vi "Generarea si afisarea grafica simultana a mai multor semnale.vi"() -> ()   [LabVIEW 2011]
uses:
  <vilib>/measure/NI_MABase.lvlib
panel:
  in  "Phase 2":dbl
  in  "Amplitude 2":dbl
  in  "Frequency 2":dbl
  in  "Sampling 2":cluster{"Fs":dbl, "#s":dbl}
  in  "Reset phase 2":bool
  in  "Reset phase":bool
  out "Waveform Graph":waveform(dbl)[](graph)
  out "error out":errorcluster
  in  "Sampling":cluster{"Fs":dbl, "#s":dbl}
  in  "Frequency":dbl
  in  "Amplitude":dbl
  in  "Phase":dbl
  in  "stop":bool
  out "error out 2":errorcluster
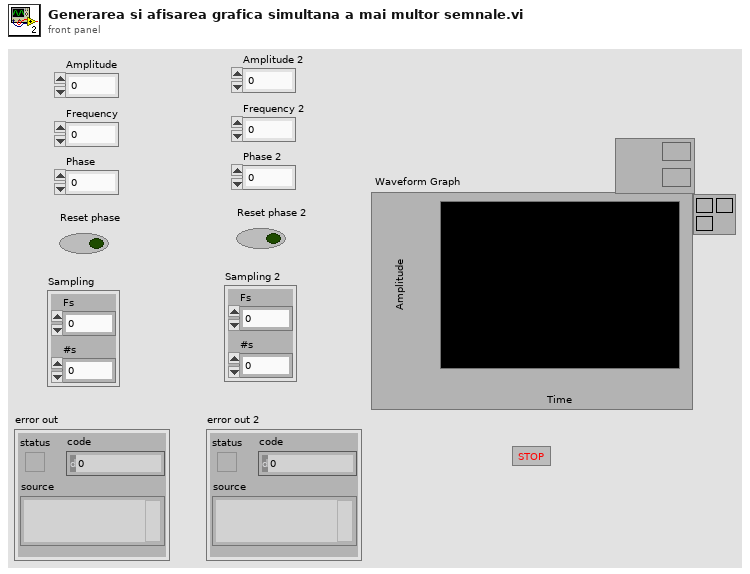
[diagram p1: front panel]
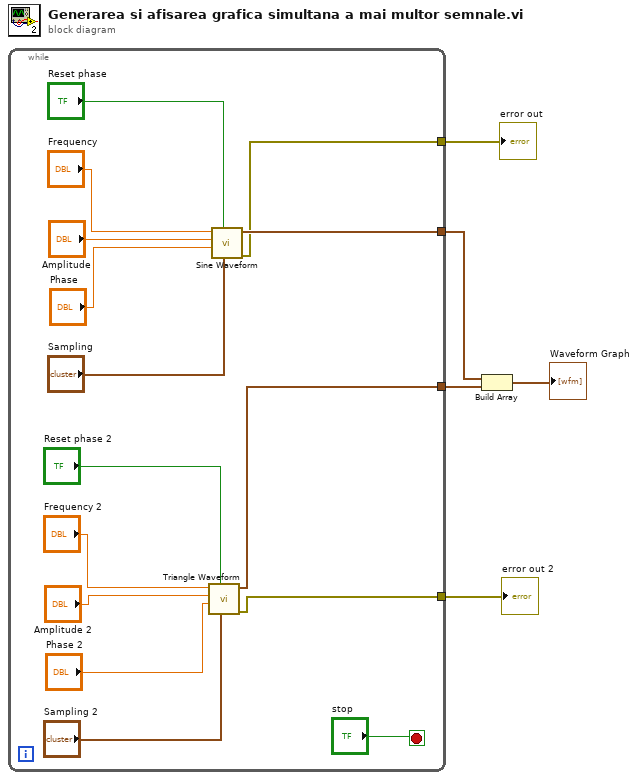
[diagram p0: block diagram]
diagram:
  n1 = while {
    tunnel: [w14] -> w5
    tunnel: [w13] -> w4
    tunnel: [w7] -> w3
    tunnel: [w6] -> w2
    stop <- "stop" stop-if-true
    n2 = call <vilib>:"Triangle Waveform.vi"("sampling info"="Sampling 2", "reset signal"="Reset phase 2", "phase"="Phase 2", "amplitude"="Amplitude 2", "frequency"="Frequency 2") -> ("error out"=w14:errorcluster, "signal out"=w13:waveform(dbl))  [unwired: 5 in]
    n3 = call <vilib>:"Sine Waveform.vi"("sampling info"="Sampling", "reset signal"="Reset phase", "phase"="Phase", "amplitude"="Amplitude", "frequency"="Frequency") -> ("error out"=w6:errorcluster, "signal out"=w7:waveform(dbl))  [unwired: 5 in]
  }
  "error out" <- w2
  "error out 2" <- w5
  n4 = Build Array(w3, w4) -> (→"Waveform Graph":waveform(dbl)[])
